vi "DDS_Clock.vi"() -> ()   [LabVIEW 2016] (continued)
"f1 [Hz] CH0"=302600000.0}, {"total time[ms]"=30.7000000000003, "f1 [Hz] CH0"=302800000.0}, {"total time[ms]"=30.7000000000003, "f1 [Hz] CH0"=302800000.0}, {"total time[ms]"=30.750000000000302, "f1 [Hz] CH0"=303000000.0}, {"total time[ms]"=30.750000000000302, "f1 [Hz] CH0"=303000000.0}, {"total time[ms]"=30.800000000000303, "f1 [Hz] CH0"=303200000.0}, {"total time[ms]"=30.800000000000303, "f1 [Hz] CH0"=303200000.0}, {"total time[ms]"=30.850000000000303, "f1 [Hz] CH0"=303400000.0}, {"total time[ms]"=30.850000000000303, "f1 [Hz] CH0"=303400000.0}, {"total time[ms]"=30.900000000000304, "f1 [Hz] CH0"=303600000.0}, {"total time[ms]"=30.900000000000304, "f1 [Hz] CH0"=303600000.0}, {"total time[ms]"=30.950000000000305, "f1 [Hz] CH0"=303800000.0}, {"total time[ms]"=30.950000000000305, "f1 [Hz] CH0"=303800000.0}, {"total time[ms]"=31.000000000000306, "f1 [Hz] CH0"=304000000.0}, {"total time[ms]"=31.000000000000306, "f1 [Hz] CH0"=304000000.0}, {"total time[ms]"=31.050000000000306, "f1 [Hz] CH0"=304200000.0}, {"total time[ms]"=31.050000000000306, "f1 [Hz] CH0"=304200000.0}, {"total time[ms]"=31.100000000000307, "f1 [Hz] CH0"=304400000.0}, {"total time[ms]"=31.100000000000307, "f1 [Hz] CH0"=304400000.0}, {"total time[ms]"=31.150000000000308, "f1 [Hz] CH0"=304600000.0}, {"total time[ms]"=31.150000000000308, "f1 [Hz] CH0"=304600000.0}, {"total time[ms]"=31.20000000000031, "f1 [Hz] CH0"=304800000.0}, {"total time[ms]"=31.20000000000031, "f1 [Hz] CH0"=304800000.0}, {"total time[ms]"=31.25000000000031, "f1 [Hz] CH0"=305000000.0}, {"total time[ms]"=31.25000000000031, "f1 [Hz] CH0"=305000000.0}, {"total time[ms]"=31.30000000000031, "f1 [Hz] CH0"=305200000.0}, {"total time[ms]"=31.30000000000031, "f1 [Hz] CH0"=305200000.0}, {"total time[ms]"=31.35000000000031, "f1 [Hz] CH0"=305400000.0}, {"total time[ms]"=31.35000000000031, "f1 [Hz] CH0"=305400000.0}, {"total time[ms]"=31.40000000000031, "f1 [Hz] CH0"=305600000.0}, {"total time[ms]"=31.40000000000031, "f1 [Hz] CH0"=305600000.0}, {"total time[ms]"=31.450000000000312, "f1 [Hz] CH0"=305800000.0}, {"total time[ms]"=31.450000000000312, "f1 [Hz] CH0"=305800000.0}, {"total time[ms]"=31.500000000000313, "f1 [Hz] CH0"=306000000.0}, {"total time[ms]"=31.500000000000313, "f1 [Hz] CH0"=306000000.0}, {"total time[ms]"=31.550000000000313, "f1 [Hz] CH0"=306200000.0}, {"total time[ms]"=31.550000000000313, "f1 [Hz] CH0"=306200000.0}, {"total time[ms]"=31.600000000000314, "f1 [Hz] CH0"=306400000.0}, {"total time[ms]"=31.600000000000314, "f1 [Hz] CH0"=306400000.0}, {"total time[ms]"=31.650000000000315, "f1 [Hz] CH0"=306600000.0}, {"total time[ms]"=31.650000000000315, "f1 [Hz] CH0"=306600000.0}, {"total time[ms]"=31.700000000000315, "f1 [Hz] CH0"=306800000.0}, {"total time[ms]"=31.700000000000315, "f1 [Hz] CH0"=306800000.0}, {"total time[ms]"=31.750000000000316, "f1 [Hz] CH0"=307000000.0}, {"total time[ms]"=31.750000000000316, "f1 [Hz] CH0"=307000000.0}, {"total time[ms]"=31.800000000000317, "f1 [Hz] CH0"=307200000.0}, {"total time[ms]"=31.800000000000317, "f1 [Hz] CH0"=307200000.0}, {"total time[ms]"=31.850000000000318, "f1 [Hz] CH0"=307400000.0}, {"total time[ms]"=31.850000000000318, "f1 [Hz] CH0"=307400000.0}, {"total time[ms]"=31.90000000000032, "f1 [Hz] CH0"=307600000.0}, {"total time[ms]"=31.90000000000032, "f1 [Hz] CH0"=307600000.0}, {"total time[ms]"=31.95000000000032, "f1 [Hz] CH0"=307800000.0}, {"total time[ms]"=31.95000000000032, "f1 [Hz] CH0"=307800000.0}, {"total time[ms]"=32.00000000000032, "f1 [Hz] CH0"=308000000.0}, {"total time[ms]"=32.00000000000032, "f1 [Hz] CH0"=308000000.0}, {"total time[ms]"=32.05000000000032, "f1 [Hz] CH0"=308200000.0}, {"total time[ms]"=32.05000000000032, "f1 [Hz] CH0"=308200000.0}, {"total time[ms]"=32.100000000000314, "f1 [Hz] CH0"=308400000.0}, {"total time[ms]"=32.100000000000314, "f1 [Hz] CH0"=308400000.0}, {"total time[ms]"=32.15000000000031, "f1 [Hz] CH0"=308600000.0}, {"total time[ms]"=32.15000000000031, "f1 [Hz] CH0"=308600000.0}, {"total time[ms]"=32.20000000000031, "f1 [Hz] CH0"=308800000.0}, {"total time[ms]"=32.20000000000031, "f1 [Hz] CH0"=308800000.0}, {"total time[ms]"=32.250000000000306, "f1 [Hz] CH0"=309000000.0}, {"total time[ms]"=32.250000000000306, "f1 [Hz] CH0"=309000000.0}, {"total time[ms]"=32.3000000000003, "f1 [Hz] CH0"=309200000.0}, {"total time[ms]"=32.3000000000003, "f1 [Hz] CH0"=309200000.0}, {"total time[ms]"=32.3500000000003, "f1 [Hz] CH0"=309400000.0}, {"total time[ms]"=32.3500000000003, "f1 [Hz] CH0"=309400000.0}, {"total time[ms]"=32.4000000000003, "f1 [Hz] CH0"=309600000.0}, {"total time[ms]"=32.4000000000003, "f1 [Hz] CH0"=309600000.0}, {"total time[ms]"=32.450000000000294, "f1 [Hz] CH0"=309800000.0}, {"total time[ms]"=32.450000000000294, "f1 [Hz] CH0"=309800000.0}, {"total time[ms]"=32.50000000000029, "f1 [Hz] CH0"=310000000.0}, {"total time[ms]"=32.50000000000029, "f1 [Hz] CH0"=310000000.0}, {"total time[ms]"=32.55000000000029, "f1 [Hz] CH0"=310200000.00000006}, {"total time[ms]"=32.55000000000029, "f1 [Hz] CH0"=310200000.00000006}, {"total time[ms]"=32.600000000000286, "f1 [Hz] CH0"=310400000.0}, {"total time[ms]"=32.600000000000286, "f1 [Hz] CH0"=310400000.0}, {"total time[ms]"=32.65000000000028, "f1 [Hz] CH0"=310600000.0}, {"total time[ms]"=32.65000000000028, "f1 [Hz] CH0"=310600000.0}, {"total time[ms]"=32.70000000000028, "f1 [Hz] CH0"=310800000.0}, {"total time[ms]"=32.70000000000028, "f1 [Hz] CH0"=310800000.0}, {"total time[ms]"=32.75000000000028, "f1 [Hz] CH0"=311000000.0}, {"total time[ms]"=32.75000000000028, "f1 [Hz] CH0"=311000000.0}, {"total time[ms]"=32.800000000000274, "f1 [Hz] CH0"=311200000.0}, {"total time[ms]"=32.800000000000274, "f1 [Hz] CH0"=311200000.0}, {"total time[ms]"=32.85000000000027, "f1 [Hz] CH0"=311400000.0}, {"total time[ms]"=32.85000000000027, "f1 [Hz] CH0"=311400000.0}, {"total time[ms]"=32.90000000000027, "f1 [Hz] CH0"=311600000.0}, {"total time[ms]"=32.90000000000027, "f1 [Hz] CH0"=311600000.0}, {"total time[ms]"=32.950000000000266, "f1 [Hz] CH0"=311800000.0}, {"total time[ms]"=32.950000000000266, "f1 [Hz] CH0"=311800000.0}, {"total time[ms]"=33.00000000000026, "f1 [Hz] CH0"=312000000.0}, {"total time[ms]"=33.00000000000026, "f1 [Hz] CH0"=312000000.0}, {"total time[ms]"=33.05000000000026, "f1 [Hz] CH0"=312200000.0}, {"total time[ms]"=33.05000000000026, "f1 [Hz] CH0"=312200000.0}, {"total time[ms]"=33.10000000000026, "f1 [Hz] CH0"=312400000.0}, {"total time[ms]"=33.10000000000026, "f1 [Hz] CH0"=312400000.0}, {"total time[ms]"=33.150000000000254, "f1 [Hz] CH0"=312600000.0}, {"total time[ms]"=33.150000000000254, "f1 [Hz] CH0"=312600000.0}, {"total time[ms]"=33.20000000000025, "f1 [Hz] CH0"=312800000.0}, {"total time[ms]"=33.20000000000025, "f1 [Hz] CH0"=312800000.0}, {"total time[ms]"=33.25000000000025, "f1 [Hz] CH0"=313000000.0}, {"total time[ms]"=33.25000000000025, "f1 [Hz] CH0"=313000000.0}, {"total time[ms]"=33.300000000000246, "f1 [Hz] CH0"=313200000.0}, {"total time[ms]"=33.300000000000246, "f1 [Hz] CH0"=313200000.0}, {"total time[ms]"=33.35000000000024, "f1 [Hz] CH0"=313400000.0}, {"total time[ms]"=33.35000000000024, "f1 [Hz] CH0"=313400000.0}, {"total time[ms]"=33.40000000000024, "f1 [Hz] CH0"=313600000.0}, {"total time[ms]"=33.40000000000024, "f1 [Hz] CH0"=313600000.0}, {"total time[ms]"=33.45000000000024, "f1 [Hz] CH0"=313800000.0}, {"total time[ms]"=33.45000000000024, "f1 [Hz] CH0"=313800000.0}, {"total time[ms]"=33.500000000000234, "f1 [Hz] CH0"=314000000.0}, {"total time[ms]"=33.500000000000234, "f1 [Hz] CH0"=314000000.0}, {"total time[ms]"=33.55000000000023, "f1 [Hz] CH0"=314200000.0}, {"total time[ms]"=33.55000000000023, "f1 [Hz] CH0"=314200000.0}, {"total time[ms]"=33.60000000000023, "f1 [Hz] CH0"=314400000.0}, {"total time[ms]"=33.60000000000023, "f1 [Hz] CH0"=314400000.0}, {"total time[ms]"=33.650000000000226, "f1 [Hz] CH0"=314600000.0}, {"total time[ms]"=33.650000000000226, "f1 [Hz] CH0"=314600000.0}, {"total time[ms]"=33.70000000000022, "f1 [Hz] CH0"=314800000.0}, {"total time[ms]"=33.70000000000022, "f1 [Hz] CH0"=314800000.0}, {"total time[ms]"=33.75000000000022, "f1 [Hz] CH0"=315000000.0}, {"total time[ms]"=33.75000000000022, "f1 [Hz] CH0"=315000000.0}, {"total time[ms]"=33.80000000000022, "f1 [Hz] CH0"=315200000.00000006}, {"total time[ms]"=33.80000000000022, "f1 [Hz] CH0"=315200000.00000006}, {"total time[ms]"=33.850000000000215, "f1 [Hz] CH0"=315400000.0}, {"total time[ms]"=33.850000000000215, "f1 [Hz] CH0"=315400000.0}, {"total time[ms]"=33.90000000000021, "f1 [Hz] CH0"=315600000.0}, {"total time[ms]"=33.90000000000021, "f1 [Hz] CH0"=315600000.0}, {"total time[ms]"=33.95000000000021, "f1 [Hz] CH0"=315800000.0}, {"total time[ms]"=33.95000000000021, "f1 [Hz] CH0"=315800000.0}, {"total time[ms]"=34.000000000000206, "f1 [Hz] CH0"=316000000.0}, {"total time[ms]"=34.000000000000206, "f1 [Hz] CH0"=316000000.0}, {"total time[ms]"=34.0500000000002, "f1 [Hz] CH0"=316200000.0}, {"total time[ms]"=34.0500000000002, "f1 [Hz] CH0"=316200000.0}, {"total time[ms]"=34.1000000000002, "f1 [Hz] CH0"=316400000.0}, {"total time[ms]"=34.1000000000002, "f1 [Hz] CH0"=316400000.0}, {"total time[ms]"=34.1500000000002, "f1 [Hz] CH0"=316600000.0}, {"total time[ms]"=34.1500000000002, "f1 [Hz] CH0"=316600000.0}, {"total time[ms]"=34.200000000000195, "f1 [Hz] CH0"=316800000.0}, {"total time[ms]"=34.200000000000195, "f1 [Hz] CH0"=316800000.0}, {"total time[ms]"=34.25000000000019, "f1 [Hz] CH0"=317000000.0}, {"total time[ms]"=34.25000000000019, "f1 [Hz] CH0"=317000000.0}, {"total time[ms]"=34.30000000000019, "f1 [Hz] CH0"=317200000.0}, {"total time[ms]"=34.30000000000019, "f1 [Hz] CH0"=317200000.0}, {"total time[ms]"=34.350000000000186, "f1 [Hz] CH0"=317400000.0}, {"total time[ms]"=34.350000000000186, "f1 [Hz] CH0"=317400000.0}, {"total time[ms]"=34.40000000000018, "f1 [Hz] CH0"=317600000.0}, {"total time[ms]"=34.40000000000018, "f1 [Hz] CH0"=317600000.0}, {"total time[ms]"=34.45000000000018, "f1 [Hz] CH0"=317800000.0}, {"total time[ms]"=34.45000000000018, "f1 [Hz] CH0"=317800000.0}, {"total time[ms]"=34.50000000000018, "f1 [Hz] CH0"=318000000.0}, {"total time[ms]"=34.50000000000018, "f1 [Hz] CH0"=318000000.0}, {"total time[ms]"=34.550000000000175, "f1 [Hz] CH0"=318200000.0}, {"total time[ms]"=34.550000000000175, "f1 [Hz] CH0"=318200000.0}, {"total time[ms]"=34.60000000000017, "f1 [Hz] CH0"=318400000.0}, {"total time[ms]"=34.60000000000017, "f1 [Hz] CH0"=318400000.0}, {"total time[ms]"=34.65000000000017, "f1 [Hz] CH0"=318600000.0}, {"total time[ms]"=34.65000000000017, "f1 [Hz] CH0"=318600000.0}, {"total time[ms]"=34.700000000000166, "f1 [Hz] CH0"=318800000.0}, {"total time[ms]"=34.700000000000166, "f1 [Hz] CH0"=318800000.0}, {"total time[ms]"=34.75000000000016, "f1 [Hz] CH0"=319000000.0}, {"total time[ms]"=34.75000000000016, "f1 [Hz] CH0"=319000000.0}, {"total time[ms]"=34.80000000000016, "f1 [Hz] CH0"=319200000.0}, {"total time[ms]"=34.80000000000016, "f1 [Hz] CH0"=319200000.0}, {"total time[ms]"=34.85000000000016, "f1 [Hz] CH0"=319400000.0}, {"total time[ms]"=34.85000000000016, "f1 [Hz] CH0"=319400000.0}, {"total time[ms]"=34.900000000000155, "f1 [Hz] CH0"=319600000.0}, {"total time[ms]"=34.900000000000155, "f1 [Hz] CH0"=319600000.0}, {"total time[ms]"=34.95000000000015, "f1 [Hz] CH0"=319800000.0}, {"total time[ms]"=34.95000000000015, "f1 [Hz] CH0"=319800000.0}, {"total time[ms]"=35.00000000000015, "f1 [Hz] CH0"=320000000.0}, {"total time[ms]"=35.00000000000015, "f1 [Hz] CH0"=320000000.0}, {"total time[ms]"=35.050000000000146, "f1 [Hz] CH0"=319800000.0}, {"total time[ms]"=35.050000000000146, "f1 [Hz] CH0"=319800000.0}, {"total time[ms]"=35.10000000000014, "f1 [Hz] CH0"=319600000.0}, {"total time[ms]"=35.10000000000014, "f1 [Hz] CH0"=319600000.0}, {"total time[ms]"=35.15000000000014, "f1 [Hz] CH0"=319400000.0}, {"total time[ms]"=35.15000000000014, "f1 [Hz] CH0"=319400000.0}, {"total time[ms]"=35.20000000000014, "f1 [Hz] CH0"=319200000.0}, {"total time[ms]"=35.20000000000014, "f1 [Hz] CH0"=319200000.0}, {"total time[ms]"=35.250000000000135, "f1 [Hz] CH0"=319000000.0}, {"total time[ms]"=35.250000000000135, "f1 [Hz] CH0"=319000000.0}, {"total time[ms]"=35.30000000000013, "f1 [Hz] CH0"=318800000.0}, {"total time[ms]"=35.30000000000013, "f1 [Hz] CH0"=318800000.0}, {"total time[ms]"=35.35000000000013, "f1 [Hz] CH0"=318600000.0}, {"total time[ms]"=35.35000000000013, "f1 [Hz] CH0"=318600000.0}, {"total time[ms]"=35.40000000000013, "f1 [Hz] CH0"=318400000.0}, {"total time[ms]"=35.40000000000013, "f1 [Hz] CH0"=318400000.0}, {"total time[ms]"=35.450000000000124, "f1 [Hz] CH0"=318200000.0}, {"total time[ms]"=35.450000000000124, "f1 [Hz] CH0"=318200000.0}, {"total time[ms]"=35.50000000000012, "f1 [Hz] CH0"=318000000.0}, {"total time[ms]"=35.50000000000012, "f1 [Hz] CH0"=318000000.0}, {"total time[ms]"=35.55000000000012, "f1 [Hz] CH0"=317800000.0}, {"total time[ms]"=35.55000000000012, "f1 [Hz] CH0"=317800000.0}, {"total time[ms]"=35.600000000000115, "f1 [Hz] CH0"=317600000.0}, {"total time[ms]"=35.600000000000115, "f1 [Hz] CH0"=317600000.0}, {"total time[ms]"=35.65000000000011, "f1 [Hz] CH0"=317400000.0}, {"total time[ms]"=35.65000000000011, "f1 [Hz] CH0"=317400000.0}, {"total time[ms]"=35.70000000000011, "f1 [Hz] CH0"=317200000.0}, {"total time[ms]"=35.70000000000011, "f1 [Hz] CH0"=317200000.0}, {"total time[ms]"=35.75000000000011, "f1 [Hz] CH0"=317000000.0}, {"total time[ms]"=35.75000000000011, "f1 [Hz] CH0"=317000000.0}, {"total time[ms]"=35.800000000000104, "f1 [Hz] CH0"=316800000.0}, {"total time[ms]"=35.800000000000104, "f1 [Hz] CH0"=316800000.0}, {"total time[ms]"=35.8500000000001, "f1 [Hz] CH0"=316600000.0}, {"total time[ms]"=35.8500000000001, "f1 [Hz] CH0"=316600000.0}, {"total time[ms]"=35.9000000000001, "f1 [Hz] CH0"=316400000.0}, {"total time[ms]"=35.9000000000001, "f1 [Hz] CH0"=316400000.0}, {"total time[ms]"=35.950000000000095, "f1 [Hz] CH0"=316200000.0}, {"total time[ms]"=35.950000000000095, "f1 [Hz] CH0"=316200000.0}, {"total time[ms]"=36.00000000000009, "f1 [Hz] CH0"=316000000.0}, {"total time[ms]"=36.00000000000009, "f1 [Hz] CH0"=316000000.0}, {"total time[ms]"=36.05000000000009, "f1 [Hz] CH0"=315800000.0}, {"total time[ms]"=36.05000000000009, "f1 [Hz] CH0"=315800000.0}, {"total time[ms]"=36.10000000000009, "f1 [Hz] CH0"=315600000.0}, {"total time[ms]"=36.10000000000009, "f1 [Hz] CH0"=315600000.0}, {"total time[ms]"=36.150000000000084, "f1 [Hz] CH0"=315400000.0}, {"total time[ms]"=36.150000000000084, "f1 [Hz] CH0"=315400000.0}, {"total time[ms]"=36.20000000000008, "f1 [Hz] CH0"=315200000.0}, {"total time[ms]"=36.20000000000008, "f1 [Hz] CH0"=315200000.0}, {"total time[ms]"=36.25000000000008, "f1 [Hz] CH0"=315000000.0}, {"total time[ms]"=36.25000000000008, "f1 [Hz] CH0"=315000000.0}, {"total time[ms]"=36.300000000000075, "f1 [Hz] CH0"=314799999.99999994}, {"total time[ms]"=36.300000000000075, "f1 [Hz] CH0"=314799999.99999994}, {"total time[ms]"=36.35000000000007, "f1 [Hz] CH0"=314600000.0}, {"total time[ms]"=36.35000000000007, "f1 [Hz] CH0"=314600000.0}, {"total time[ms]"=36.40000000000007, "f1 [Hz] CH0"=314400000.0}, {"total time[ms]"=36.40000000000007, "f1 [Hz] CH0"=314400000.0}, {"total time[ms]"=36.45000000000007, "f1 [Hz] CH0"=314200000.0}, {"total time[ms]"=36.45000000000007, "f1 [Hz] CH0"=314200000.0}, {"total time[ms]"=36.500000000000064, "f1 [Hz] CH0"=314000000.0}, {"total time[ms]"=36.500000000000064, "f1 [Hz] CH0"=314000000.0}, {"total time[ms]"=36.55000000000006, "f1 [Hz] CH0"=313800000.0}, {"total time[ms]"=36.55000000000006, "f1 [Hz] CH0"=313800000.0}, {"total time[ms]"=36.60000000000006, "f1 [Hz] CH0"=313600000.0}, {"total time[ms]"=36.60000000000006, "f1 [Hz] CH0"=313600000.0}, {"total time[ms]"=36.650000000000055, "f1 [Hz] CH0"=313400000.0}, {"total time[ms]"=36.650000000000055, "f1 [Hz] CH0"=313400000.0}, {"total time[ms]"=36.70000000000005, "f1 [Hz] CH0"=313200000.0}, {"total time[ms]"=36.70000000000005, "f1 [Hz] CH0"=313200000.0}, {"total time[ms]"=36.75000000000005, "f1 [Hz] CH0"=313000000.0}, {"total time[ms]"=36.75000000000005, "f1 [Hz] CH0"=313000000.0}, {"total time[ms]"=36.80000000000005, "f1 [Hz] CH0"=312800000.0}, {"total time[ms]"=36.80000000000005, "f1 [Hz] CH0"=312800000.0}, {"total time[ms]"=36.850000000000044, "f1 [Hz] CH0"=312600000.0}, {"total time[ms]"=36.850000000000044, "f1 [Hz] CH0"=312600000.0}, {"total time[ms]"=36.90000000000004, "f1 [Hz] CH0"=312400000.0}, {"total time[ms]"=36.90000000000004, "f1 [Hz] CH0"=312400000.0}, {"total time[ms]"=36.95000000000004, "f1 [Hz] CH0"=312200000.0}, {"total time[ms]"=36.95000000000004, "f1 [Hz] CH0"=312200000.0}, {"total time[ms]"=37.000000000000036, "f1 [Hz] CH0"=312000000.0}, {"total time[ms]"=37.000000000000036, "f1 [Hz] CH0"=312000000.0}, {"total time[ms]"=37.05000000000003, "f1 [Hz] CH0"=311800000.0}, {"total time[ms]"=37.05000000000003, "f1 [Hz] CH0"=311800000.0}, {"total time[ms]"=37.10000000000003, "f1 [Hz] CH0"=311600000.0}, {"total time[ms]"=37.10000000000003, "f1 [Hz] CH0"=311600000.0}, {"total time[ms]"=37.15000000000003, "f1 [Hz] CH0"=311400000.0}, {"total time[ms]"=37.15000000000003, "f1 [Hz] CH0"=311400000.0}, {"total time[ms]"=37.200000000000024, "f1 [Hz] CH0"=311200000.0}, {"total time[ms]"=37.200000000000024, "f1 [Hz] CH0"=311200000.0}, {"total time[ms]"=37.25000000000002, "f1 [Hz] CH0"=311000000.0}, {"total time[ms]"=37.25000000000002, "f1 [Hz] CH0"=311000000.0}, {"total time[ms]"=37.30000000000002, "f1 [Hz] CH0"=310800000.0}, {"total time[ms]"=37.30000000000002, "f1 [Hz] CH0"=310800000.0}, {"total time[ms]"=37.350000000000016, "f1 [Hz] CH0"=310600000.0}, {"total time[ms]"=37.350000000000016, "f1 [Hz] CH0"=310600000.0}, {"total time[ms]"=37.40000000000001, "f1 [Hz] CH0"=310400000.0}, {"total time[ms]"=37.40000000000001, "f1 [Hz] CH0"=310400000.0}, {"total time[ms]"=37.45000000000001, "f1 [Hz] CH0"=310200000.0}, {"total time[ms]"=37.45000000000001, "f1 [Hz] CH0"=310200000.0}, {"total time[ms]"=37.50000000000001, "f1 [Hz] CH0"=310000000.0}, {"total time[ms]"=37.50000000000001, "f1 [Hz] CH0"=310000000.0}, {"total time[ms]"=37.550000000000004, "f1 [Hz] CH0"=309799999.99999994}, {"total time[ms]"=37.550000000000004, "f1 [Hz] CH0"=309799999.99999994}, {"total time[ms]"=37.6, "f1 [Hz] CH0"=309600000.0}, {"total time[ms]"=37.6, "f1 [Hz] CH0"=309600000.0}, {"total time[ms]"=37.65, "f1 [Hz] CH0"=309400000.0}, {"total time[ms]"=37.65, "f1 [Hz] CH0"=309400000.0}, {"total time[ms]"=37.699999999999996, "f1 [Hz] CH0"=309200000.0}, {"total time[ms]"=37.699999999999996, "f1 [Hz] CH0"=309200000.0}, {"total time[ms]"=37.74999999999999, "f1 [Hz] CH0"=309000000.0}, {"total time[ms]"=37.74999999999999, "f1 [Hz] CH0"=309000000.0}, {"total time[ms]"=37.79999999999999, "f1 [Hz] CH0"=308800000.0}, {"total time[ms]"=37.79999999999999, "f1 [Hz] CH0"=308800000.0}, {"total time[ms]"=37.84999999999999, "f1 [Hz] CH0"=308600000.0}, {"total time[ms]"=37.84999999999999, "f1 [Hz] CH0"=308600000.0}, {"total time[ms]"=37.899999999999984, "f1 [Hz] CH0"=308400000.0}, {"total time[ms]"=37.899999999999984, "f1 [Hz] CH0"=308400000.0}, {"total time[ms]"=37.94999999999998, "f1 [Hz] CH0"=308200000.0}, {"total time[ms]"=37.94999999999998, "f1 [Hz] CH0"=308200000.0}, {"total time[ms]"=37.99999999999998, "f1 [Hz] CH0"=308000000.0}, {"total time[ms]"=37.99999999999998, "f1 [Hz] CH0"=308000000.0}, {"total time[ms]"=38.049999999999976, "f1 [Hz] CH0"=307800000.0}, {"total time[ms]"=38.049999999999976, "f1 [Hz] CH0"=307800000.0}, {"total time[ms]"=38.09999999999997, "f1 [Hz] CH0"=307600000.0}, {"total time[ms]"=38.09999999999997, "f1 [Hz] CH0"=307600000.0}, {"total time[ms]"=38.14999999999997, "f1 [Hz] CH0"=307400000.0}, {"total time[ms]"=38.14999999999997, "f1 [Hz] CH0"=307400000.0}, {"total time[ms]"=38.19999999999997, "f1 [Hz] CH0"=307200000.0}, {"total time[ms]"=38.19999999999997, "f1 [Hz] CH0"=307200000.0}, {"total time[ms]"=38.249999999999964, "f1 [Hz] CH0"=307000000.0}, {"total time[ms]"=38.249999999999964, "f1 [Hz] CH0"=307000000.0}, {"total time[ms]"=38.29999999999996, "f1 [Hz] CH0"=306800000.0}, {"total time[ms]"=38.29999999999996, 
